vi "subvi_movingpieces.vi"(4 "Upper White Row":i32, 5 "solved puzzle":picture[][](array[picture]), 7 "current puzzle state":picture[][](array[picture]), 8 "Current Selected Peice Column":i32, 9 "Current Selected Peice Row":i32, 10 "Lower White  Column":i32, 11 "Allow Peice Movement":bool) -> (2 "Puzzle Finished":bool, 3 "updated image array":picture[][](array[picture]))   [LabVIEW 2014]
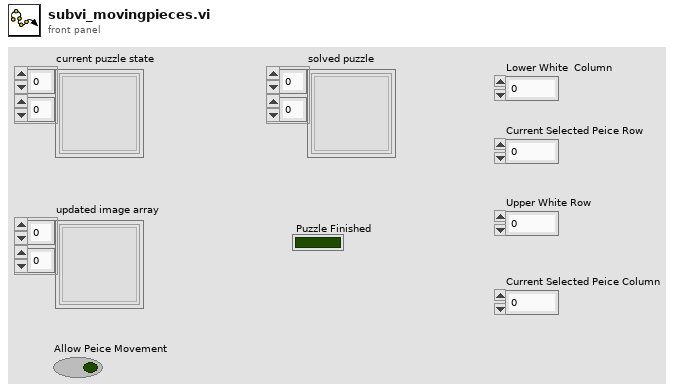
[diagram p1: front panel]
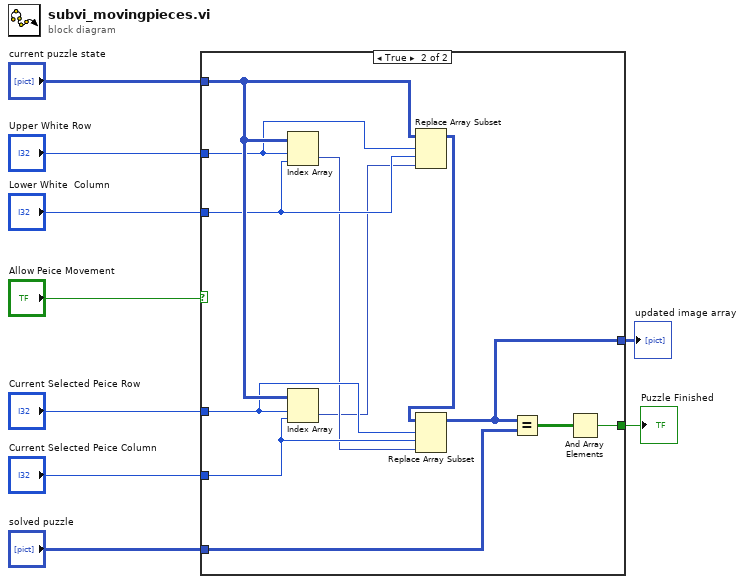
[diagram p0: block diagram]
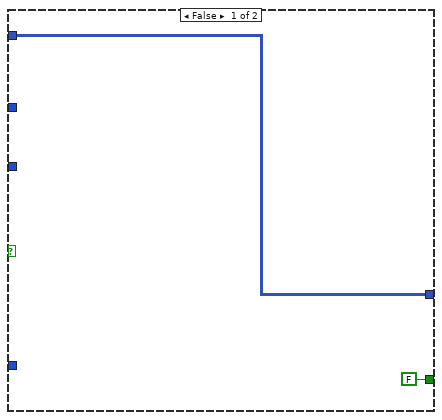
[diagram p2: hidden frame]
diagram:
  n1 = case shown="True" "Allow Peice Movement" {
    tunnel: "Upper White Row" -> [_ w14]
    tunnel: "current puzzle state" -> [w11 w23]
    tunnel: "solved puzzle" -> [_ w21]
    tunnel: [FALSE w19] -> w5
    tunnel: "Current Selected Peice Row" -> [_ w18]
    tunnel: "Lower White  Column" -> [_ w17]
    tunnel: "Current Selected Peice Column" -> [_ w16]
    tunnel: [w11 w15] -> w1
    frame False {
    }
    frame True {
      n2 = Index Array(array=w23, index (row)=w14, index (col)=w17) -> (element=w13:picture)
      n3 = Index Array(array=w23, index (row)=w18, index (col)=w16) -> (element=w12:picture)
      n4 = Replace Array Subset(array=w23, new element=w12, index (row)=w14, index (col)=w17) -> (w22:picture[][])
      n5 = Replace Array Subset(array=w22, new element=w13, index (row)=w18, index (col)=w16) -> (w15:picture[][])
      n6 = Equal?(x=w15, y=w21) -> (x = y?=w20:bool[][])
      n7 = And Array Elements(Boolean array=w20) -> (logical AND=w19:bool)
    }
  }
  "Puzzle Finished" <- w5
  "updated image array" <- w1
